vi "Drive Controller.vi"(8 "error in":errorcluster) -> ()   [LabVIEW 2016]
doc: "This VI executes continuously carrying out the current operation and responding to updates or new operation requests. It will often contain the timing or control code that is difficult to place directly in TeleOp. This VI generally opens all sensors and motors and isolates the rest of the robot code from knowing implementation details of how the operations are carried out."
uses:
  Drive Operations.ctl
  Drive Setpoints.ctl
  <vilib>/Rock Robotics/WPI/SafetyOutput/WPI_SafetyOutputConfigMenu.ctl
  <vilib>/Rock Robotics/WPI/ThirdParty/CanMotor/TalonSRX/WPI_CANTalonSRX_APIControlMode.ctl
  <vilib>/Rock Robotics/WPI/Solenoid/WPI_SolenoidChannel.ctl
  <vilib>/Rock Robotics/WPI/Counter/WPI_CounterDigitalInputToDigitalSource.vi
  <vilib>/Rock Robotics/SystemInterfaces/DIO/FPGA_DIOChannel.ctl
  <vilib>/platform/TimedLoop/XDataNode/XDataNode.xnode
  <vilib>/Platform/TimedLoop/XDataNode/nitl_modes.ctl
  <vilib>/Platform/TimedLoop/XDataNode/XDNodeRunTimeDep.lvlib
  <vilib>/Platform/TimedLoop/XDataNode/wakeup.ctl
  <vilib>/Platform/TimedLoop/XDataNode/timing_clust.ctl
  <vilib>/Rock Robotics/WPI/Solenoid/WPI_SolenoidValue.ctl
  <vilib>/Rock Robotics/WPI/Solenoid/WPI_SolenoidSetEnum.vi
  <vilib>/addons/control/pid/NI_PID_pid.lvlib
  <vilib>/addons/control/pid/pid.llb/PID (DBL).vi
  <vilib>/Rock Robotics/WPI/Solenoid/WPI_SolenoidOpenDouble.vi
  <vilib>/Rock Robotics/WPI/RobotDrive/WPI_RobotDriveOpen2MotorWithExistingMotors.vi
  <vilib>/Rock Robotics/WPI/ThirdParty/Sensors/Pigeon IMU/CTRE_PigeonIMU_Open_CAN.vi
panel:
  in  "PID gains Right Velocity":T1={"proportional gain (Kc)"=1.0, "integral time (Ti, min)"=0.01, "derivative time (Td, min)"=0.0} {"derivative time (Td, min)" format="%.3f"; "integral time (Ti, min)" format="%.3f"; "proportional gain (Kc)" format="%.3f"}
  in  "PID gains Left Velocity":T1={"proportional gain (Kc)"=1.0, "integral time (Ti, min)"=0.01, "derivative time (Td, min)"=0.0} {"derivative time (Td, min)" format="%.3f"; "integral time (Ti, min)" format="%.3f"; "proportional gain (Kc)" format="%.3f"}
  out "Instantaneous Right Velocity (ft/s)":dbl
  out "Instantaneous Left Velocity (ft/s)":dbl
  out "YPR Yaw":dbl
  in  "PID gains":T1={"proportional gain (Kc)"=1.0, "integral time (Ti, min)"=0.01, "derivative time (Td, min)"=0.0} {"derivative time (Td, min)" format="%.3f"; "integral time (Ti, min)" format="%.3f"; "proportional gain (Kc)" format="%.3f"}
  in  "scale":dbl=0.4
  in  "ticks/rev":dbl=512.0 format="%#_13g"
  out "Accelerration (ft/s2)":T2(graph)
  out "Velocity (ft/s)":T2(graph)
  out "Setpoints":T2(graph)
  out "Current\nCmd":string
  # "Tip: It may be helpful to observe inputs and sensor values.\nYou may also want to display tuning or debugging controls."
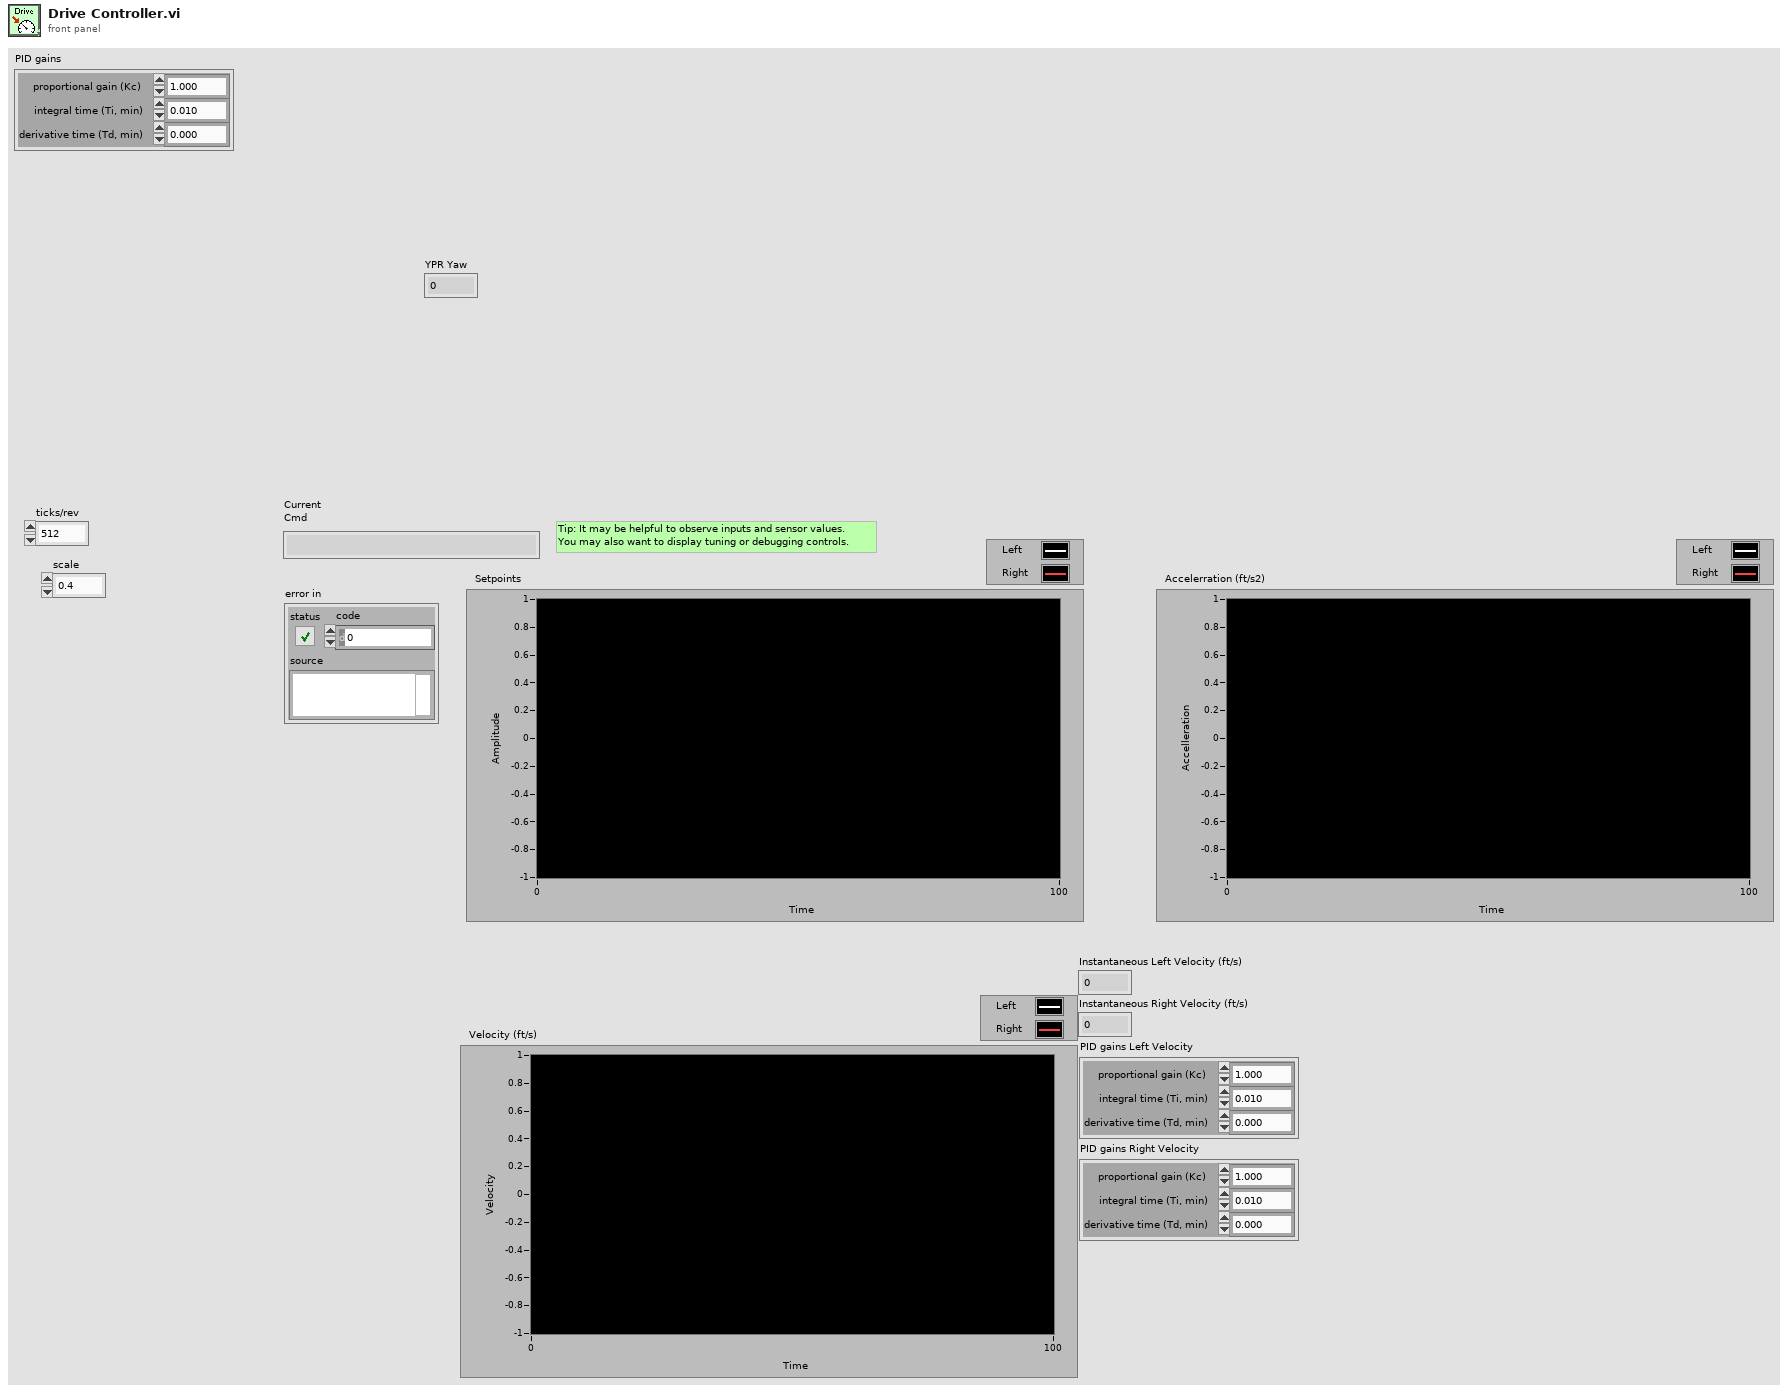
[diagram p1: front panel]
types:
  T1 = cluster{"proportional gain (Kc)":dbl, "integral time (Ti, min)":dbl, "derivative time (Td, min)":dbl}
  T2 = cluster{"Left Setpoint":dbl, "Right Setpoint":dbl}
  T3 = typedef "FPGA_DIOChannel.ctl" = enum8{"DIO 0", "DIO 1", "DIO 2", "DIO 3", "DIO 4", "DIO 5", "DIO 6", "DIO 7", "DIO 8", "DIO 9", "DIO MXP 0", "DIO MXP 1", "DIO MXP 2", "DIO MXP 3", "DIO MXP 4", "DIO MXP 5", "DIO MXP 6", "DIO MXP 7", "DIO MXP 8", "DIO MXP 9", "DIO MXP 10", "DIO MXP 11", "DIO MXP 12", "DIO MXP 13", "DIO MXP 14", "DIO MXP 15", "SPI Port CS1", "SPI Port CS2", "SPI Port CS3", "SPI Port MISO", "SPI Port MOSI", "Invalid"}
  T4 = typedef "WPI_SolenoidChannel.ctl" = enum8{"Solenoid 0", "Solenoid 1", "Solenoid 2", "Solenoid 3", "Solenoid 4", "Solenoid 5", "Solenoid 6", "Solenoid 7", "Invalid"}
  T5 = typedef "WPI_CANTalonSRX_APIControlMode.ctl" = enum8{"Percent VBus", "Speed", "Position", "Slave", "Unchanged / Invalid", "Voltage Compensation", "Current", "Motion Profile", "Motion Magic"}
  T6 = typedef "WPI_SafetyOutputConfigMenu.ctl" = enum16{"Enable", "Disable"}
  T7 = typedef "Drive Setpoints.ctl" = cluster{"Operation":T8, "Left Setpoint":dbl, "Right Setpoint":dbl, "Duration (time)":dbl, "Shift State":i32, "Distance":dbl, "Angle":dbl}
  T8 = typedef "Drive Operations.ctl" = enum16{"Reserve", "Velocity Control", "Read Current", "Drive a Curve", "Turn to Angle", "Immediate", "Drive for Time", "Drive for Distance"}
  T9 = typedef "WPI_MotorControlDeviceRef.ctl" = cluster{"DeviceStatus":errorcluster, "Type":T10, "PWM":cluster{"PWM Channel":T11, "DeadBand":T12}, "CAN":cluster{"Device Number":u8, "SetOutput VI Ref":variant, "GetOutput VI Ref":variant, "Enable VI Ref":variant, "Disable VI Ref":variant, "Data":variant}, "Invert":bool}
  T10 = typedef "WPI_MotorControlType.ctl" = enum16{"PWM", "CAN"}
  T11 = typedef "FPGA_DIOPWMChannel.ctl" = enum8{"PWM 0", "PWM 1", "PWM 2", "PWM 3", "PWM 4", "PWM 5", "PWM 6", "PWM 7", "PWM 8", "PWM 9", "PWM MXP 0", "PWM MXP 1", "PWM MXP 2", "PWM MXP 3", "PWM MXP 4", "PWM MXP 5", "PWM MXP 6", "PWM MXP 7", "PWM MXP 8", "PWM MXP 9", "Invalid"}
  T12 = typedef "WPI_PWMDeadband.ctl" = cluster{"Name":string, "maxPositivePwm":i32, "minPositivePwm":i32, "centerPwm":i32, "maxNegativePwm":i32, "minNegativePwm":i32, "angularRange":u16}
  T13 = typedef "WPI_RobotDriveDevRef.ctl" = cluster{"DevStatus":errorcluster, "Motors[]":T9[], "Square Inputs":bool, "Max Output":dbl}
  T14 = typedef "WPI_DigitalInputDevRef.ctl" = cluster{"DevStatus":errorcluster, "DIO Channel":T3}
  T15 = typedef "FPGA_CounterEncoderSourceConvertionLVSourceType.ctl" = cluster{"DevStatus":errorcluster, "AnalogTriggerMode?":bool, "DigitalMode":cluster{"DIO Channel":T16}, "AnalogTriggerMode":cluster{"AnalogTriggerIndex":T17, "OutputType":T18}}
  T16 = typedef "FPGA_DIODigitalSourceChannel.ctl" = enum8{"DIO 0", "DIO 1", "DIO 2", "DIO 3", "DIO 4", "DIO 5", "DIO 6", "DIO 7", "DIO 8", "DIO 9", "DIO MXP 0", "DIO MXP 1", "DIO MXP 2", "DIO MXP 3", "DIO MXP 4", "DIO MXP 5", "DIO MXP 6", "DIO MXP 7", "DIO MXP 8", "DIO MXP 9", "DIO MXP 10", "DIO MXP 11", "DIO MXP 12", "DIO MXP 13", "DIO MXP 14", "DIO MXP 15", "Disabled"}
  T17 = typedef "FPGA_AnalogTriggerIndex.ctl" = enum8{"Trig 0", "Trig 1", "Trig 2", "Trig 3", "Trig 4", "Trig 5", "Trig 6", "Trig 7", "Invalid"}
  T18 = typedef "FPGA_AnalogTriggerOutType.ctl" = enum16{"InWindow", "TriggerState", "Rising", "Falling"}
  T19 = typedef "CTRE_PigeonIMU_DeviceRef.ctl" = cluster{"DeviceStatus":errorcluster, "Device Number":u8, "Type":T20, "Device ID":u32}
  T20 = typedef "CTRE_PigeonIMU_ConnectionType.ctl" = u32
  T21 = typedef "WPI_EncoderDevRef.ctl" = cluster{"DevStatus":errorcluster, "EncoderIndex":T22, "CounterIndex":T23, "DistancePerCount":dbl, "Decoding Type":T24}
  T22 = typedef "FPGA_EncoderIdx.ctl" = enum8{"Enc 0", "Enc 1", "Enc 2", "Enc 3", "Enc 4", "Enc 5", "Enc 6", "Enc 7", "Invalid"}
  T23 = typedef "FPGA_CounterCtrSystemIndex.ctl" = enum8{"Ctr 0", "Ctr 1", "Ctr 2", "Ctr 3", "Ctr 4", "Ctr 5", "Ctr 6", "Ctr 7", "Invalid"}
  T24 = typedef "WPI_EncoderType.ctl" = enum16{"1x", "2x", "4x"}
  T25 = typedef "Command Status Info.ctl" = cluster{"Name":string, "Status":T26, "notifier out":T27}
  T26 = typedef "Completion Status.ctl" = enum16{"Successful", "Aborted", "Incomplete"}
  T27 = typedef "Completion Notifier.ctl" = refnum<notifier>
  T28 = cluster{"SubSystem Data":T7, cluster{"Start Time (ms)":u32, "Iterations":i32}, cluster{"Command Info":T25, "Description":string, "SubSystem Data":T7, "notifier out":refnum<notifier>, "Subsystem Name":string}}
  T29 = typedef "WPI_SolenoidDevRef.ctl" = cluster{"DevStatus":errorcluster, "Pneumatics Control Module":u8, "Forward Solenoid Channel":T4, "Reverse Solenoid Channel":T4}
  T30 = typedef "CTRE_PigeonIMU_GlobalStatus.ctl" = cluster{"PigeonState":T31, "FusedHeading":cluster{"Heading":dbl, "Valid?":bool, "Fusing?":bool}, "YPR":cluster{"Yaw":dbl, "Pitch":dbl, "Roll":dbl}, "Compass":cluster{"Heading":dbl, "Magnitude":dbl, "Absolute Heading":dbl}, "Accelerometer":cluster{"Biased":cluster{"X":i16, "Y":i16, "Z":i16, "Norm":i16}, "Angles":cluster{"XZ Tilt":dbl, "YZ Tilt":dbl, "XY Tilt":dbl}}, "Magnetometer":cluster{"Raw":cluster{"X":i16, "Y":i16, "Z":i16}, "Biased":cluster{"X":i16, "Y":i16, "Z":i16}}, "Gyro":cluster{"X":dbl, "Y":dbl, "Z":dbl, "Norm":dbl}, "6D Quaternian":cluster{"W":dbl, "X":dbl, "Y":dbl, "Z":dbl}, "Temp. (C)":dbl, "UpTime":u32, "StartupStatus":cluster{"ResetCount":i32, "ResetFlags":i32, "FirmwareVersion":i32, "HasReset?":bool}, "Calibration":cluster{"CurrentMode":T32, "LastCalError":i32, "CalBooting?":bool}, "CAN Error":errorcluster, "AccumGyro":cluster{"X":dbl, "Y":dbl, "Z":dbl}, "Usage Frame":u32}
  T31 = typedef "CTRE_PigeonIMU_PigeonState.ctl" = enum16{"NoComm", "Initializing", "Ready", "UserCalibration"}
  T32 = typedef "CTRE_PigeonIMU_CalibrationMode.ctl" = u16
  T33 = typedef "WPI_SolenoidValue.ctl" = enum16{"Off", "On", "Forward", "Reverse"}
  T34 = cluster{"SubSystem Data":T7, cluster{"Start Time (ms)":u32, "Iterations":i32}, "Default Command Arguments":cluster{"Command Info":T25, "Description":string, "SubSystem Data":T7, "notifier out":refnum<notifier>, "Subsystem Name":string}}
  T35 = cluster{"Don't move motors while reserved":dbl, "Don't move motors while reserved":dbl}
  T36 = typedef "XDNodeRunTimeDep.lvlib/timing_clust.ctl" = cluster{"Expected End [f-1]":u64, "Actual End [f-1]":u64, "Finished Late? [f-1]":bool, "Expected End [i-1]":u64, "Actual End [i-1]":u64, "Finished Late? [i-1]":bool, "Expected Start [i]":u64, "Actual Start [i]":u64, "Expected Start [f]":u64, "Actual Start [f]":u64, "Source Name":string, "Structure Name":string, "Period":i64, "Deadline":i64, "Offset":i64, "Start":i64, "Priority":i32, "Timeout":i32, "Mode":T37, "Wakeup Reason":T38, "Error":errorcluster, "Source Type":string, "Secondary Source Type":string, "Global End Time":u64, "Global Start Time":u64, "Frame Duration":u64, "Iteration Duration":u64, "Assigned CPU":i32, "I/O Scan Engine Mode":u32}
  T37 = typedef "XDNodeRunTimeDep.lvlib/nitl_modes.ctl" = enum32{"No Change", "Process missed periods, maintain original phase", "Discard missed periods, maintain original phase", "Process missed periods, ignore original phase", "Discard missed periods, ignore original phase"}
  T38 = typedef "XDNodeRunTimeDep.lvlib/wakeup.ctl" = enum32{"Normal", "Aborted", "Asynchronous wakeup", "Timing source error", "Timed loop error", "Timeout"}
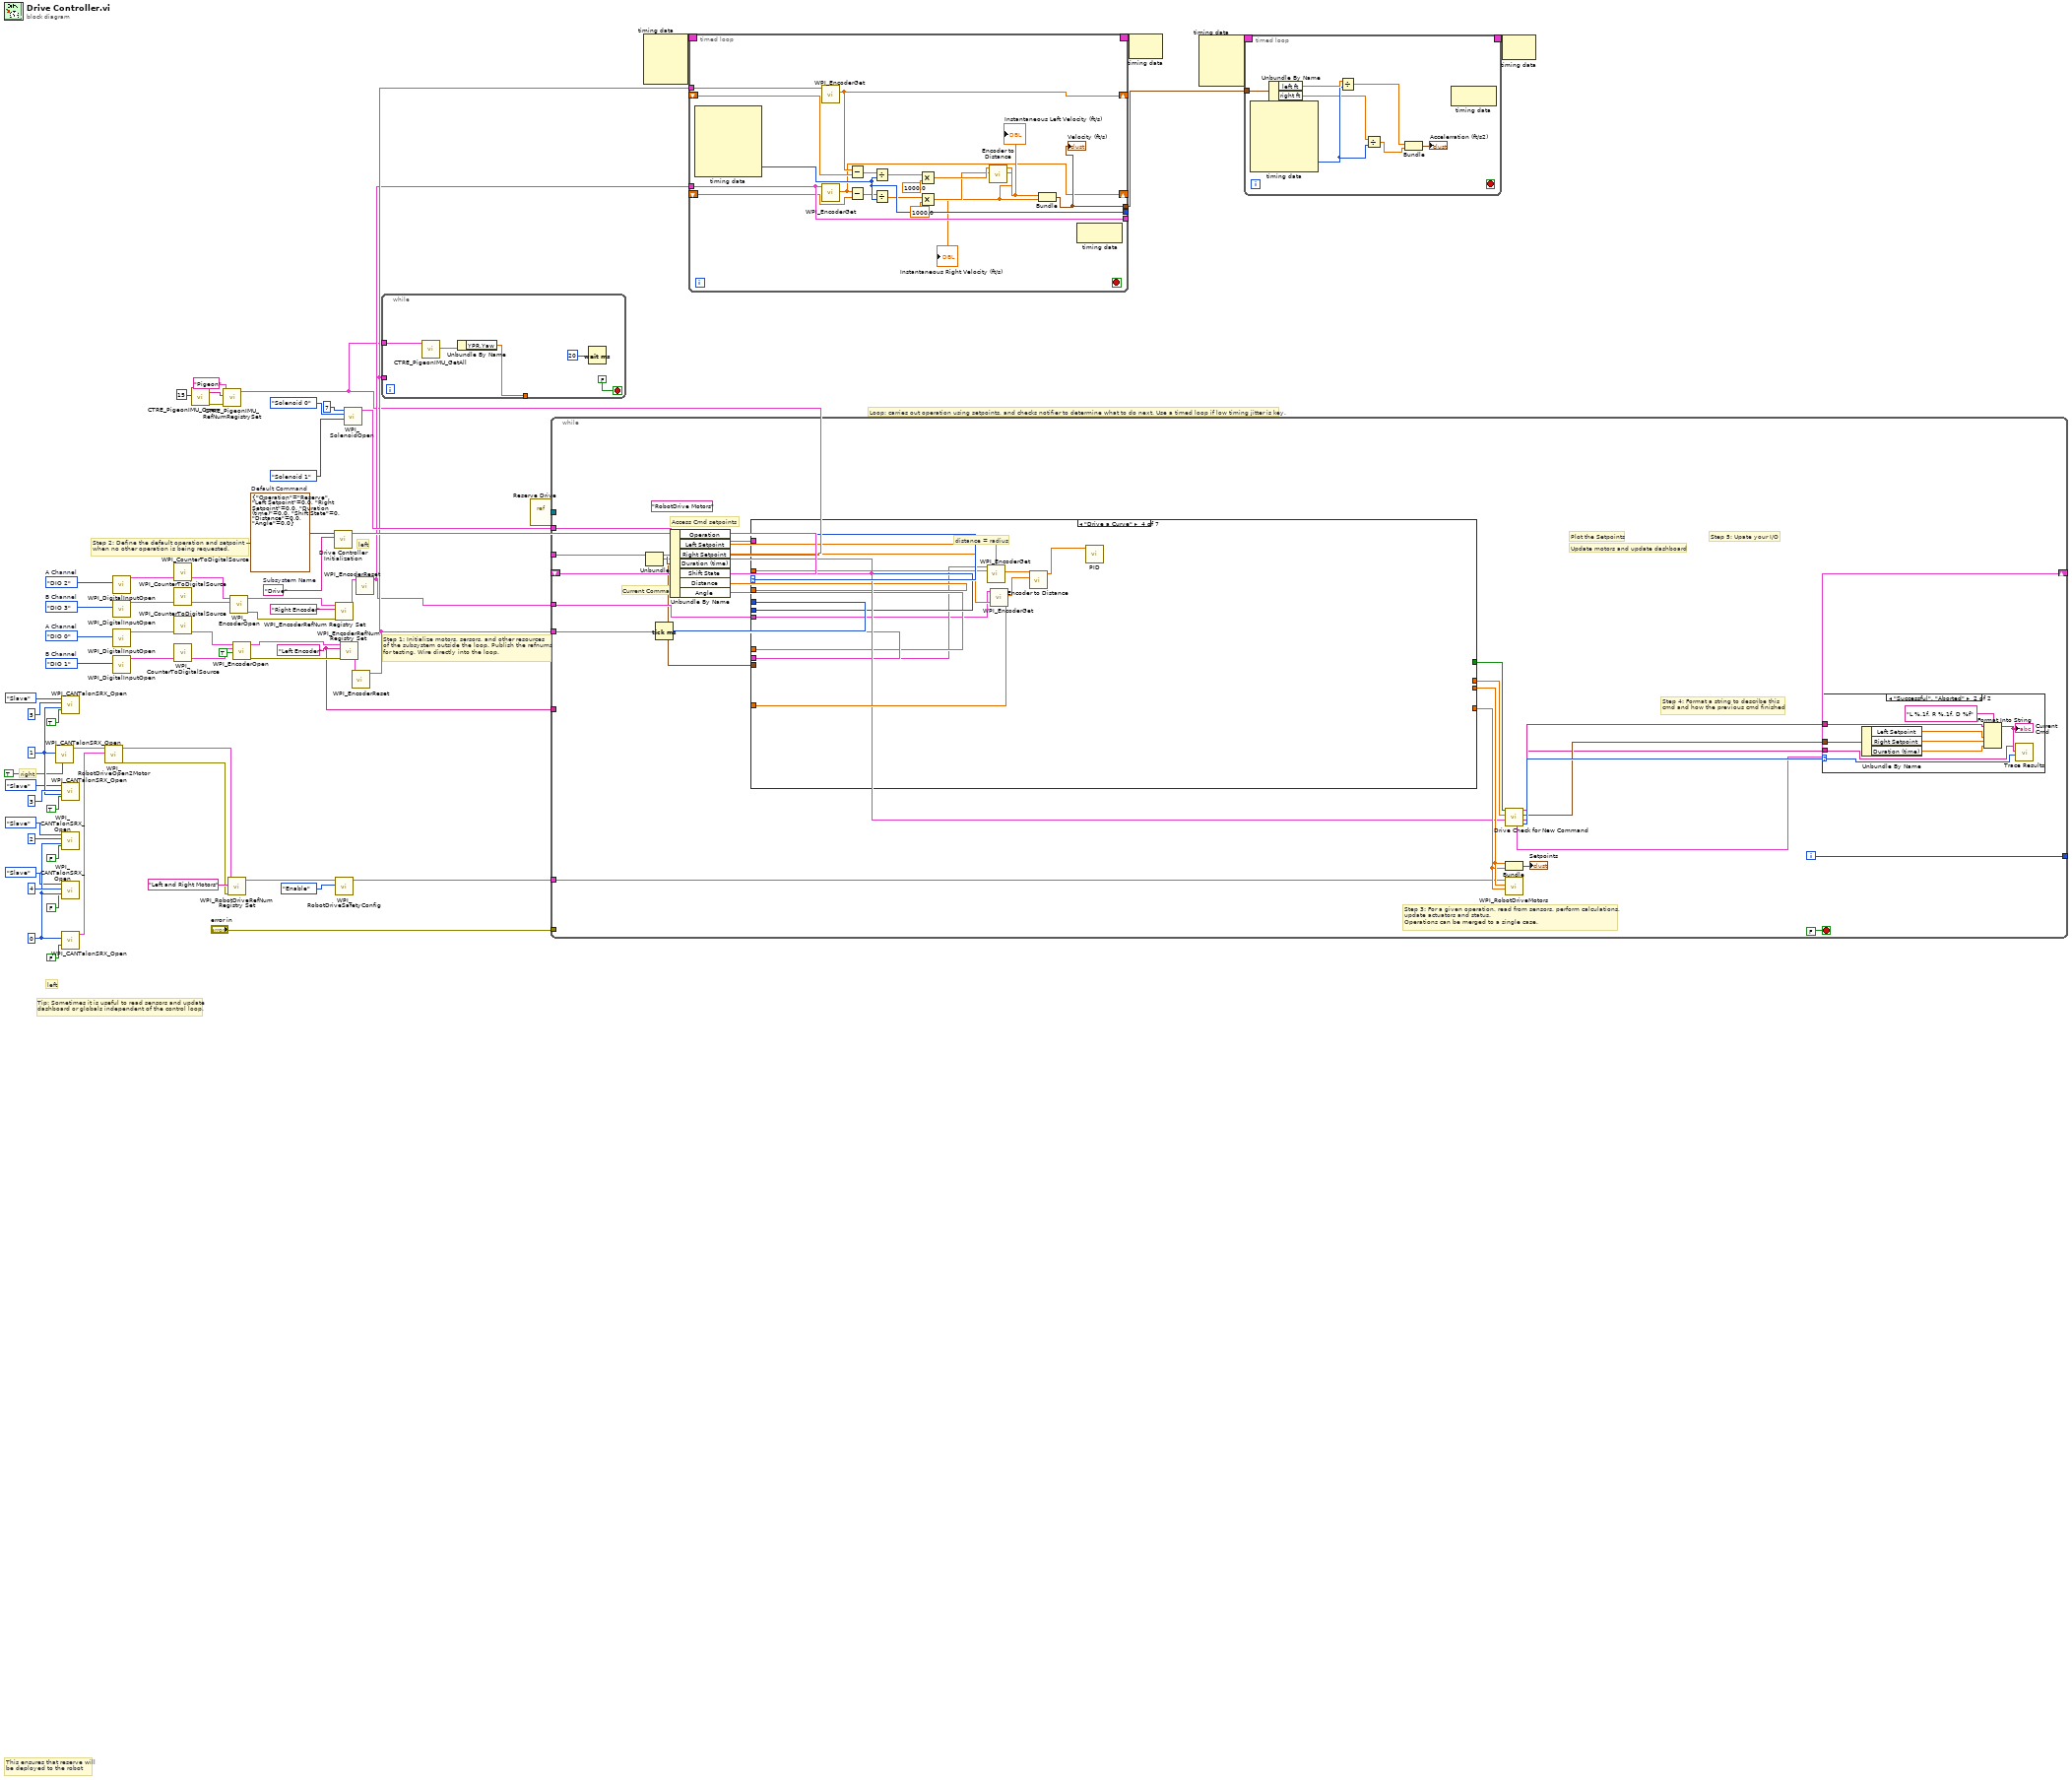
[diagram p0: block diagram]
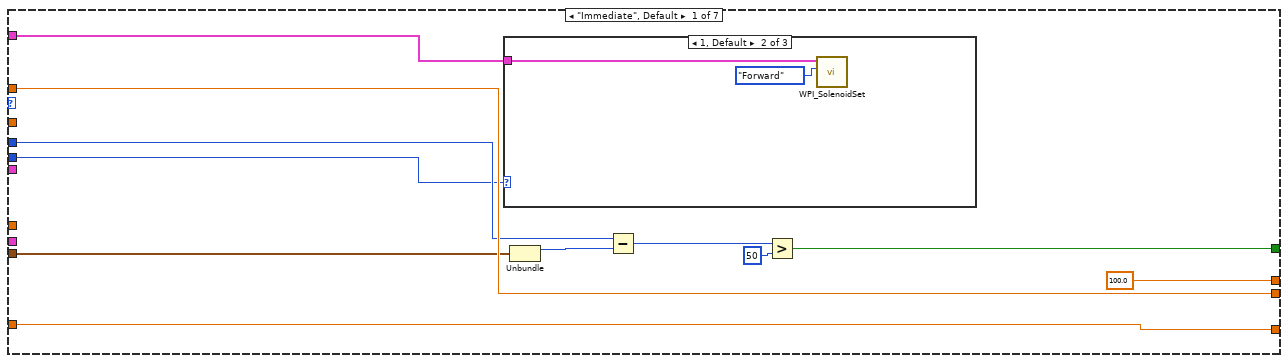
[diagram p3: hidden frame]
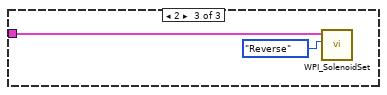
[diagram p5: hidden frame]
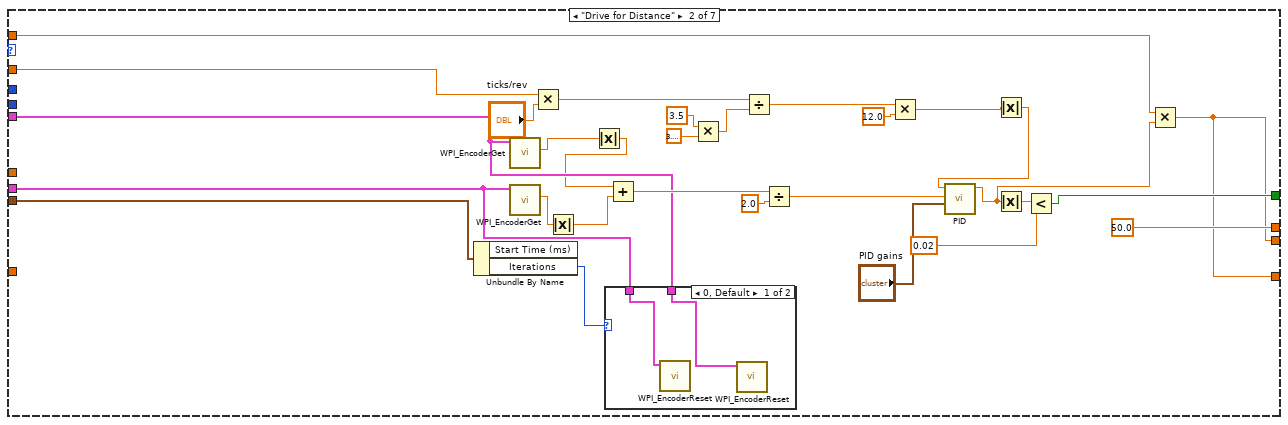
[diagram p6: hidden frame]
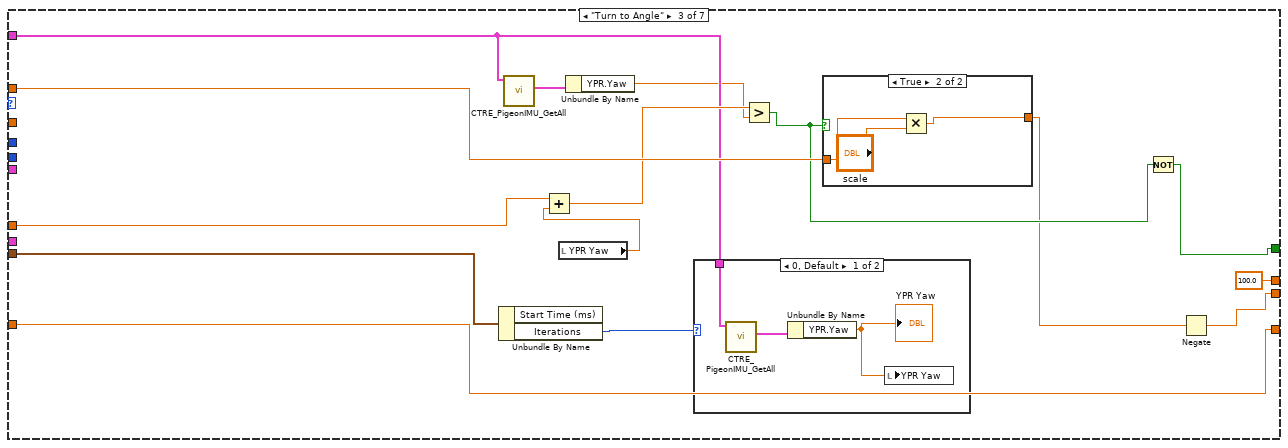
[diagram p8: hidden frame]
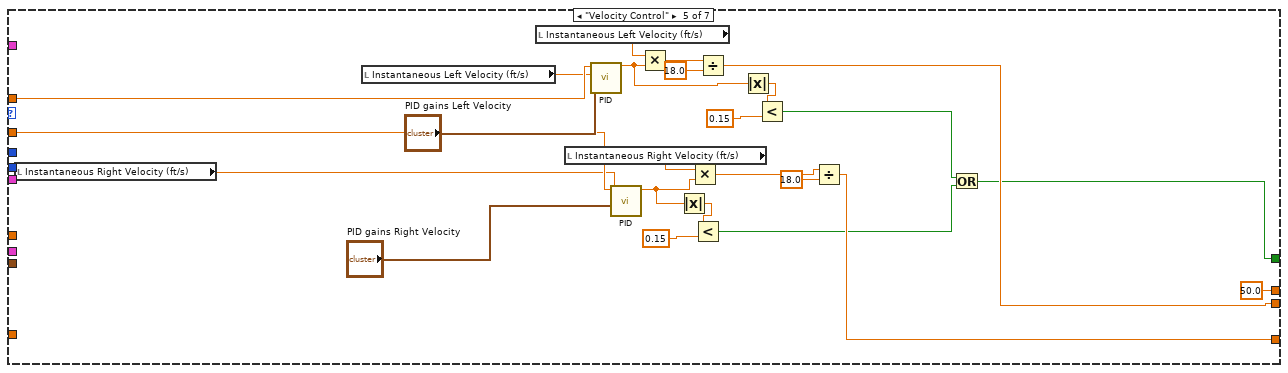
[diagram p11: hidden frame]
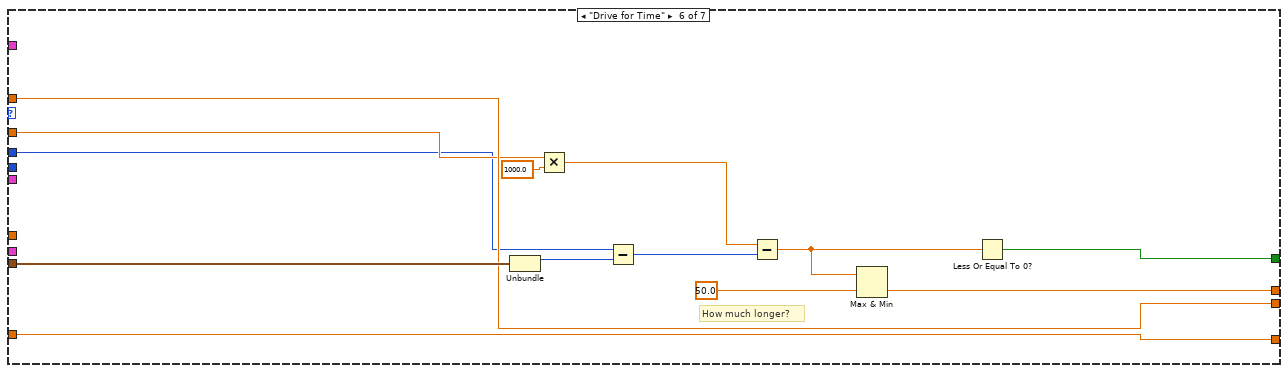
[diagram p12: hidden frame]
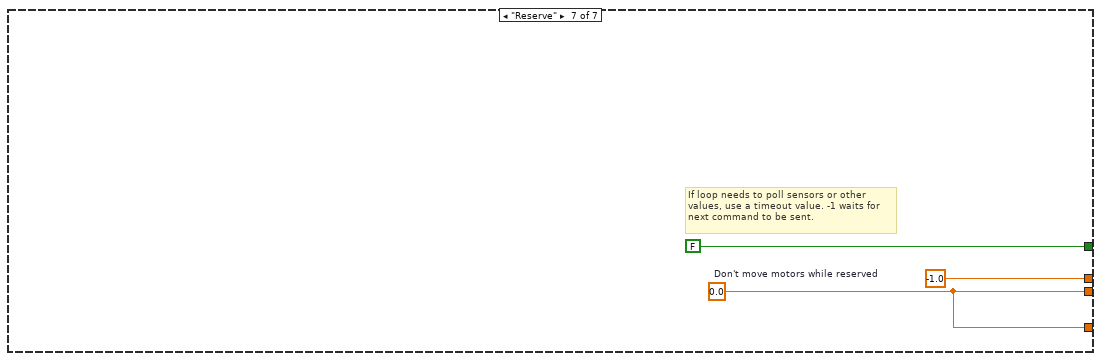
[diagram p13: hidden frame]
diagram:
  w6 = "Left Encoder" ("refnum name")
  w30 = FPGA_DIOChannel."DIO 1"  # B Channel
  w29 = FPGA_DIOChannel."DIO 0"  # A Channel
  w36 = FPGA_DIOChannel."DIO 3"  # B Channel
  w35 = FPGA_DIOChannel."DIO 2"  # A Channel
  w49 = u8 1 ("Device Number")
  w46 = u8 0 ("Device Number")
  w65 = T7 {"Operation"=enum."Reserve", "Left Setpoint"=0.0, "Right Setpoint"=0.0, "Duration (time)"=0.0, "Shift State"=0, "Distance"=0.0, "Angle"=0.0}  # Default Command
  w66 = "Drive"  # Subsystem Name
  # "left"
  # "right"
  # "left"
  # "This ensures that reserve will\nbe deployed to the robot"
  # "Tip: Sometimes it is useful to read sensors and update\ndashboard or globals independent of the control loop."
  # "Step 2: Define the default operation and setpoint --\nwhen no other operation is being requested."
  # "Step 1: Initialize motors, sersors, and other resources\nof the subsystem outside the loop. Publish the refnums\nfor testing. Wire directly into the loop."
  # "Loop: carries out operation using setpoints, and checks notifier to determine what to do next. Use a timed loop if low timing jitter is key."
  n1 = call <vilib>:"WPI_CANTalonSRX_Open.vi"("Invert"=TRUE, "Device Number"=w49) -> ("CAN Talon SRX Ref"=w55:T9)  [unwired: 8 in, 1 out]
  n2 = call <vilib>:"WPI_CANTalonSRX_Open.vi"("Invert"=TRUE, "Master Device Number"=w49, "Device Number"=u8 5, "Control Mode"=WPI_CANTalonSRX_APIControlMode."Slave") -> ()  [unwired: 6 in, 2 out]
  n3 = call <vilib>:"WPI_CANTalonSRX_Open.vi"("Invert"=TRUE, "Master Device Number"=w49, "Device Number"=u8 3, "Control Mode"=WPI_CANTalonSRX_APIControlMode."Slave") -> ()  [unwired: 6 in, 2 out]
  n4 = call <vilib>:"WPI_CANTalonSRX_Open.vi"("Invert"=FALSE, "Master Device Number"=w46, "Device Number"=u8 2, "Control Mode"=WPI_CANTalonSRX_APIControlMode."Slave") -> ()  [unwired: 6 in, 2 out]
  n5 = call <vilib>:"WPI_CANTalonSRX_Open.vi"("Invert"=FALSE, "Master Device Number"=w46, "Device Number"=u8 4, "Control Mode"=WPI_CANTalonSRX_APIControlMode."Slave") -> ()  [unwired: 6 in, 2 out]
  n6 = call <vilib>:"WPI_CANTalonSRX_Open.vi"("Invert"=FALSE, "Device Number"=w46) -> ("CAN Talon SRX Ref"=w54:T9)  [unwired: 8 in, 1 out]
  n7 = call-poly <vilib>:"WPI_RobotDriveOpen2Motor.vi"("Right Motor Dev Ref"=w54, "Left Motor Dev Ref"=w55) -> ("error out"=w62:errorcluster, "RobotDriveDevRef"=w64:T13)  [unwired: 3 in, 5 out]
  n8 = call <vilib>:"WPI_DigitalInputOpen.vi"("DIO Channel"=w35) -> ("DigitalInputDevRef"=w32:T14)  [unwired: 1 in, 9 out]
  n9 = call <vilib>:"WPI_DigitalInputOpen.vi"("DIO Channel"=w36) -> ("DigitalInputDevRef"=w33:T14)  [unwired: 1 in, 9 out]
  n10 = call <vilib>:"WPI_DigitalInputOpen.vi"("DIO Channel"=w29) -> ("DigitalInputDevRef"=w26:T14)  [unwired: 1 in, 9 out]
  n11 = call <vilib>:"WPI_DigitalInputOpen.vi"("DIO Channel"=w30) -> ("DigitalInputDevRef"=w27:T14)  [unwired: 1 in, 9 out]
  n12 = call-poly <vilib>:"WPI_CounterToDigitalSource.vi"("DigitalInputDevRef"=w32) -> ("Digital Source"=w31:T15)  [unwired: 6 out]
  n13 = call-poly <vilib>:"WPI_CounterToDigitalSource.vi"("DigitalInputDevRef"=w33) -> ("Digital Source"=w34:T15)  [unwired: 6 out]
  n14 = call-poly <vilib>:"WPI_CounterToDigitalSource.vi"("DigitalInputDevRef"=w26) -> ("Digital Source"=w25:T15)  [unwired: 6 out]
  n15 = call-poly <vilib>:"WPI_CounterToDigitalSource.vi"("DigitalInputDevRef"=w27) -> ("Digital Source"=w28:T15)  [unwired: 6 out]
  n16 = call-poly <vilib>:"CTRE_PigeonIMU_Open.vi"("Device Number"=u8 15) -> ("error out"=w5:errorcluster, "PigeonIMUDevRef"=w4:T19)  [unwired: 9 in]
  n17 = call <vilib>:"CTRE_PigeonIMU_RefNumRegistrySet.vi"("error in (no error)"=w5, "refnum name"="Pigeon", "PigeonIMUDevRef"=w4) -> ("PigeonIMUDevRef"=w1:T19)  [unwired: 7 in, 1 out]
  n18 = call <vilib>:"WPI_RobotDriveRefNum Registry Set.vi"("error in (no error)"=w62, "refnum name"="Left and Right Motors", "RobotDriveDevRef"=w64) -> ("RobotDriveDevRef"=w61:T13)  [unwired: 1 in, 7 out]
  n19 = call <vilib>:"WPI_EncoderOpen.vi"("BSource"=w34, "ASource"=w31) -> ("error out"=w24:errorcluster, "EncoderDevRef"=w23:T21)  [unwired: 6 in, 2 out]
  n20 = call <vilib>:"WPI_EncoderOpen.vi"("Invert Direction (False)"=TRUE, "BSource"=w28, "ASource"=w25) -> ("error out"=w21:errorcluster, "EncoderDevRef"=w22:T21)  [unwired: 5 in, 2 out]
  n21 = call "Drive Controller Initialization.vi"("Subsystem Name"=w66, "Default Command"=w65) -> ("output cluster"=w57:T28)  [unwired: 9 in]
  n22 = call <vilib>:"WPI_EncoderRefNum Registry Set.vi"("error in (no error)"=w24, "refnum name"="Right Encoder", "EncoderDevRef"=w23) -> ("EncoderDevRef"=w9:T21)  [unwired: 7 in, 1 out]
  n23 = call <vilib>:"WPI_RobotDriveSafetyConfig.vi"("mode"=WPI_SafetyOutputConfigMenu."Enable", "RobotDriveDevRef"=w61) -> ("RobotDriveDevRef"=w59:T13)  [unwired: 8 in, 1 out]
  n24 = call <vilib>:"WPI_EncoderRefNum Registry Set.vi"("error in (no error)"=w21, "refnum name"=w6, "EncoderDevRef"=w22) -> ("EncoderDevRef"=w11:T21)  [unwired: 7 in, 1 out]
  n25 = call-poly <vilib>:"WPI_SolenoidOpen.vi"("Reverse Solenoid Channel"=WPI_SolenoidChannel."Solenoid 1", "Forward Solenoid Channel"=WPI_SolenoidChannel."Solenoid 0", "Pneumatics Control Module (0)"=u8 7) -> ("SolenoidDevRef"=w37:T29)  [unwired: 7 in, 1 out]
  n26 = call <vilib>:"WPI_EncoderReset.vi"("EncoderDevRef"=w11) -> ("EncoderDevRef"=w10:T21)  [unwired: 9 in, 1 out]
  n27 = call <vilib>:"WPI_EncoderReset.vi"("EncoderDevRef"=w9) -> ("EncoderDevRef"=w8:T21)  [unwired: 9 in, 1 out]
  n28 = while {
    tunnel: w10 -> [_]
    tunnel: w1 -> [w68]
    tunnel: [w67] -> _
    stop <- FALSE stop-if-true
    n29 = call <vilib>:"CTRE_PigeonIMU_GetAll.vi"("PigeonIMUDevRef"=w68) -> ("Get All"=w69:T30)  [unwired: 8 in, 2 out]
    n30 = Unbundle By Name(w69) -> ("YPR.Yaw"=w67:dbl)
    n31 = Wait (ms)(milliseconds to wait=u32 20) -> ()  [unwired: 1 out]
  }
  n32 = vi-ref "Reserve Drive.vi"() -> (w56:refnum<vi>)
  n33 = while {
    shift-right: [w86] -> _
    shift-left: w57 -> [w80]
    tunnel: [w96] -> _
    tunnel: w59 -> [w93]
    tunnel: "error in" -> [_]
    tunnel: w56 -> [_]
    tunnel: w37 -> [w72]
    tunnel: w8 -> [w78]
    tunnel: w10 -> [w77]
    tunnel: w6 -> [_]
    tunnel: w1 -> [_]
    i -> [w96]
    stop <- FALSE stop-if-true
    (unwired) "RobotDrive Motors" ("Name")
    # "Step 5: Upate your I/O"
    # "Step 4: Format a string to describe this\ncmd and how the previous cmd finished"
    # "Current Command"
    # "Update motors and update dashboard"
    # "Plot the Setpoints"
    # "Access Cmd setpoints"
    # "Step 3: For a given operation, read from sensors, perform calculations,\nupdate actuators and status.\nOperations can be merged to a single case."
    n34 = Unbundle(w80) -> ("SubSystem Data"=w92:T7, w73:cluster{"Start Time (ms)":u32, "Iterations":i32})  [unwired: 1 out]
    n35 = Tick Count (ms)() -> (millisecond timer value=w88:u32)
    n36 = Unbundle By Name(w92) -> ("Operation"=w91:T8, "Left Setpoint"=w90:dbl, "Right Setpoint"=w89:dbl, "Shift State"=w79:i32, "Distance"=w74:dbl, "Angle"=w75:dbl)  [unwired: 1 out]
    n37 = case shown="\"Drive a Curve\"" w91 {
      tunnel: [100.0 50.0 100.0 _ 50.0 w204 -1.0] -> w85
      tunnel: [w110 w125 w162 _ w180 w211 FALSE ("ignore previous (F)")] -> w84
      tunnel: w73 -> [w109 w139 w156 _ _ w213 _]
      tunnel: [w116 w122 w160 _ w190 w210 w217] -> w95
      tunnel: [w115 w122 w165 _ w189 w209 w217] -> w94
      tunnel: w90 -> [w116 w123 w166 _ w203 w210 _]
      tunnel: w89 -> [w115 _ w165 _ _ w209 _]
      tunnel: w74 -> [_ w141 _ _ w200 w208 _]
      tunnel: w88 -> [w111 _ _ _ _ w207 _]
      tunnel: w79 -> [w108 _ _ _ _ _ _]
      tunnel: w72 -> [w107 _ w154 _ _ _ _]
      tunnel: w78 -> [_ w136 _ w177 _ _ _]
      tunnel: w77 -> [_ w137 _ w179 _ _ _]
      tunnel: w75 -> [_ _ w159 _ _ _ _]
      frame "Immediate", Default {
        n38 = case shown="1, Default" w108 {
          tunnel: w107 -> [_ w119 w120]
          frame 0 {
          }
          frame 1, Default {
            n39 = call-poly <vilib>:"WPI_SolenoidSet.vi"("Value"=WPI_SolenoidValue."Forward", "SolenoidDevRef"=w119) -> ()  [unwired: 8 in, 2 out]
          }
          frame 2 {
            n40 = call-poly <vilib>:"WPI_SolenoidSet.vi"("Value"=WPI_SolenoidValue."Reverse", "SolenoidDevRef"=w120) -> ()  [unwired: 8 in, 2 out]
          }
        }
        n41 = Unbundle(w109) -> ("Start Time (ms)"=w112:u32)  [unwired: 1 out]
        n42 = Subtract(x=w111, y=w112) -> (x-y=w113:u32)
        n43 = Greater?(x=w113, y=u8 50 ("Left Motor")) -> (0:w110:bool)
      }
      frame "Drive for Distance" {
        n44 = Unbundle By Name(w139) -> ("Iterations"=w138:i32)  [unwired: 1 out]
        n45 = call <vilib>:"WPI_EncoderGet.vi"("EncoderDevRef"=w136) -> ("Distance"=w132:dbl)  [unwired: 5 in, 5 out]
        n46 = call <vilib>:"WPI_EncoderGet.vi"("EncoderDevRef"=w137) -> ("Distance"=w134:dbl)  [unwired: 5 in, 5 out]
        n47 = Multiply(x=w141, y="ticks/rev") -> (x*y=w147:dbl)
        n48 = Absolute Value(x=w134) -> (abs(x)=w133:dbl)
        n49 = Absolute Value(x=w132) -> (abs(x)=w131:dbl)
        n50 = case shown="0, Default" w138 {
          tunnel: w137 -> [w152 _]
          tunnel: w136 -> [w151 _]
          frame 0, Default {
            n51 = call <vilib>:"WPI_EncoderReset.vi"("EncoderDevRef"=w152) -> ()  [unwired: 9 in, 2 out]
            n52 = call <vilib>:"WPI_EncoderReset.vi"("EncoderDevRef"=w151) -> ()  [unwired: 9 in, 2 out]
          }
          frame 1 {
          }
        }
        n53 = Add(x=w131, y=w133) -> (x+y=w150:dbl)
        n54 = Multiply(x=3.5 ("y"), y=3.141592653589793) -> (x*y=w145:dbl)
        n55 = Divide(x=w147, y=w145) -> (x/y=w143:dbl)
        n56 = Divide(x=w150, y=2.0) -> (x/y=w129:dbl)
        n57 = Multiply(x=w143, y=12.0) -> (x*y=w135:dbl)
        n58 = Absolute Value(x=w135) -> (abs(x)=w130:dbl)
        n59 = call-poly <vilib>:"PID.vi"("PID gains"="PID gains", "process variable"=w129, "setpoint"=w130) -> ("output"=w124:dbl)  [unwired: 7 in, 1 out]
        n60 = Absolute Value(x=w124) -> (abs(x)=w127:dbl)
        n61 = Less?(x=w127, y=0.02) -> (x < y?=w125:bool)
        n62 = Multiply(x=w123, y=w124) -> (x*y=w122:dbl)
      }
      frame "Turn to Angle" {
        n63 = Unbundle By Name(w156) -> ("Iterations"=w155:i32)  [unwired: 1 out]
        n64 = call <vilib>:"CTRE_PigeonIMU_GetAll.vi"("PigeonIMUDevRef"=w154) -> ("Get All"=w167:T30)  [unwired: 8 in, 2 out]
        n65 = local read "YPR Yaw"() -> (w157:dbl)
        n66 = Add(x=w159, y=w157) -> (x+y=w158:dbl)
        n67 = Unbundle By Name(w167) -> ("YPR.Yaw"=w153:dbl)
        n68 = case shown="0, Default" w155 {
          tunnel: w154 -> [w169 _]
          frame 0, Default {
            n69 = call <vilib>:"CTRE_PigeonIMU_GetAll.vi"("PigeonIMUDevRef"=w169) -> ("Get All"=w170:T30)  [unwired: 8 in, 2 out]
            n70 = Unbundle By Name(w170) -> ("YPR.Yaw"=w168:dbl)
            "YPR Yaw" <- w168
            n71 = local write "YPR Yaw"(w168) -> ()
          }
          frame 1 {
          }
        }
        n72 = Greater?(x=w158, y=w153) -> (0:w163:bool)
        n73 = case shown="True" w163 {
          tunnel: w166 -> [w171 w174]
          tunnel: [w171 w172] -> w161
          frame False {
          }
          frame True {
            n74 = Multiply(x=w174, y="scale") -> (x*y=w172:dbl)
          }
        }
        n75 = Not(x=w163) -> (.not. x?=w162:bool)
        n76 = Negate(x=w161) -> (-x=w160:dbl)
      }
      frame "Drive a Curve" {
        # "distance = radius"
        n77 = call <vilib>:"WPI_EncoderGet.vi"("EncoderDevRef"=w179) -> ("Distance"=w178:dbl)  [unwired: 5 in, 5 out]
        n78 = call <vilib>:"WPI_EncoderGet.vi"("EncoderDevRef"=w177) -> ("Distance"=w176:dbl)  [unwired: 5 in, 5 out]
        n79 = call "Encoder to Distance.vi"("Right Encoder"=w176, "Left Encoder"=w178) -> ("left ft"=w175:dbl)  [unwired: 8 in, 1 out]
        n80 = call-poly <vilib>:"PID.vi"("setpoint"=w175) -> ()  [unwired: 9 in, 2 out]
      }
      frame "Velocity Control" {
        n81 = local read "Instantaneous Right Velocity (ft/s)"() -> (w199:dbl)
        n82 = local read "Instantaneous Left Velocity (ft/s)"() -> (w202:dbl)
        n83 = local read "Instantaneous Left Velocity (ft/s)"() -> (w194:dbl)
        n84 = local read "Instantaneous Right Velocity (ft/s)"() -> (w197:dbl)
        n85 = call-poly <vilib>:"PID.vi"("PID gains"="PID gains Left Velocity", "process variable"=w202, "setpoint"=w203) -> ("output"=w184:dbl)  [unwired: 7 in, 1 out]
        n86 = call-poly <vilib>:"PID.vi"("PID gains"="PID gains Right Velocity", "process variable"=w199, "setpoint"=w200) -> ("output"=w187:dbl)  [unwired: 7 in, 1 out]
        n87 = Multiply(x=w194, y=w184) -> (x*y=w193:dbl)
        n88 = Absolute Value(x=w187) -> (abs(x)=w186:dbl)
        n89 = Multiply(x=w197, y=w187) -> (x*y=w196:dbl)
        n90 = Less?(x=w186, y=0.15) -> (x < y?=w181:bool)
        n91 = Divide(x=w193, y=18.0) -> (x/y=w190:dbl)
        n92 = Absolute Value(x=w184) -> (abs(x)=w183:dbl)
        n93 = Less?(x=w183, y=0.15) -> (x < y?=w182:bool)
        n94 = Divide(x=w196, y=18.0) -> (x/y=w189:dbl)
        n95 = Or(x=w182, y=w181) -> (x .or. y?=w180:bool)
      }
      frame "Drive for Time" {
        # "How much longer?"
        n96 = Unbundle(w213) -> ("Start Time (ms)"=w212:u32)  [unwired: 1 out]
        n97 = Multiply(x=w208, y=1000.0) -> (x*y=w215:dbl)
        n98 = Subtract(x=w207, y=w212) -> (x-y=w216:u32)
        n99 = Subtract(x=w215, y=w216) -> (x-y=w206:dbl)
        n100 = Max & Min(x=w206, y=50.0) -> (min(x,y)=w204:dbl)  [unwired: 1 out]
        n101 = Less Or Equal To 0?(x=w206) -> (x <= 0?=w211:bool)
      }
      frame "Reserve" {
        w217 = 0.0  # Don't move motors while reserved
        # "If loop needs to poll sensors or other\nvalues, use a timeout value. -1 waits for\nnext command to be sent."
      }
    }
    n102 = call "Drive Check for New Command.vi"("input cluster"=w80, "Wait time (ms)"=w85, "Finished?"=w84) -> ("Completion"=w87:T26, "Subsystem Name"=w81:string, "SetPoint"=w82:T7, "Initial Trace String"=w83:string, "output cluster"=w86:T34)  [unwired: 4 in]
    n103 = Bundle("Don't move motors while reserved"=w95, "Don't move motors while reserved"=w94) -> (→"Setpoints":T35)  [unwired: 1 in]
    n104 = call <vilib>:"WPI_RobotDriveMotors.vi"("RightSpeed"=w94, "LeftSpeed"=w95, "RobotDriveDevRef"=w93) -> ()  [unwired: 1 in, 8 out]
    n105 = case shown="\"Successful\", \"Aborted\"" w87 {
      selector: w87 -> [_ w106]
      tunnel: w83 -> [_ w101]
      tunnel: w82 -> [_ w102]
      tunnel: w81 -> [_ w98]
      frame "Incomplete", Default {
        # "Continuing current command"
      }
      frame "Successful", "Aborted" {
        # "Report and setup for next command"
        n106 = Unbundle By Name(w102) -> ("Left Setpoint"=w104:dbl, "Right Setpoint"=w105:dbl, "Duration (time)"=w99:dbl)
        n107 = Format Into String(format string="L %.1f, R %.1f, D %f", initial string=w101, w104, w105, w99) -> (resulting string=w100:string)  [unwired: 1 in, 1 out]
        "Current\nCmd" <- w100
        n108 = call <vilib>:"Trace Results.vi"("Status of previous command"=w106, "Description"=w100, "Subsystem"=w98) -> ()  [unwired: 9 in]
      }
    }
  }
  n109 = node-c288() -> (w19:T36)  [unwired: 4 in]
  n110 = timed-loop {
    timing: w19 -> [_]
    timing-out: [_] -> w18
    tunnel: [w237] -> _
    tunnel: w8 -> [w237]
    tunnel: w10 -> [w236]
    tunnel: [w235] -> _
    shift-right: [w220] -> _
    shift-left: _ -> [w228]
    shift-right: [w230] -> _
    shift-left: _ -> [w229]
    tunnel: [w221] -> w15
    stop <- _ stop-if-true
    n111 = node-c288() -> (w235:i64)  [unwired: 1 in, 6 out]
    n112 = call <vilib>:"WPI_EncoderGet.vi"("EncoderDevRef"=w236) -> ("Distance"=w230:dbl)  [unwired: 5 in, 5 out]
    n113 = call <vilib>:"WPI_EncoderGet.vi"("EncoderDevRef"=w237) -> ("Distance"=w220:dbl)  [unwired: 5 in, 5 out]
    n114 = Subtract(x=w230, y=w229) -> (x-y=w231:dbl)
    n115 = Subtract(x=w220, y=w228) -> (x-y=w232:dbl)
    n116 = Divide(x=w231, y=w235) -> (x/y=w227:dbl)
    n117 = Divide(x=w232, y=w235) -> (x/y=w226:dbl)
    n118 = Multiply(x=w227, y=1000.0) -> (x*y=w225:dbl)
    n119 = Multiply(x=w226, y=1000.0) -> (x*y=w224:dbl)
    n120 = call "Encoder to Distance.vi"("Right Encoder"=w224, "Left Encoder"=w225) -> ("right ft"=w222:dbl, "left ft"=w223:dbl)  [unwired: 8 in]
    "Instantaneous Left Velocity (ft/s)" <- w223
    "Instantaneous Right Velocity (ft/s)" <- w222
    n121 = Bundle("left ft"=w223, "right ft"=w222) -> (w221:cluster{"left ft":dbl, "right ft":dbl})  [unwired: 1 in]
    "Velocity (ft/s)" <- w221
    n122 = node-c288() -> ()  [unwired: 1 in, 1 out]
  }
  n123 = node-c288(w18) -> ()  [unwired: 1 out]
  n124 = node-c288() -> (w17:T36)  [unwired: 4 in]
  n125 = timed-loop {
    timing: w17 -> [_]
    timing-out: [_] -> w16
    tunnel: w15 -> [w247]
    stop <- _ stop-if-true
    n126 = node-c288() -> (w245:i64)  [unwired: 1 in, 6 out]
    n127 = Unbundle By Name(w247) -> ("left ft"=w246:dbl, "right ft"=w244:dbl)
    n128 = Divide(x=w246, y=w245) -> (x/y=w242:dbl)
    n129 = Divide(x=w244, y=w245) -> (x/y=w241:dbl)
    n130 = Bundle(w242, w241) -> (→"Accelerration (ft/s2)":cluster{dbl, dbl})  [unwired: 1 in]
    n131 = node-c288() -> ()  [unwired: 1 in, 1 out]
  }
  n132 = node-c288(w16) -> ()  [unwired: 1 out]
